vi "Converter.vi"() -> ()   [LabVIEW 2017]
uses:
  CodeElements/SetReturnValue_class/SetReturnValue.lvclass
  E:/Code_Generator/CodeElements/Base/CodeElement.lvclass
  CodeElements/Base/CodeElement.lvclass
panel:
  out "Header":string
  out "Execution":string
  in  "vi path":path
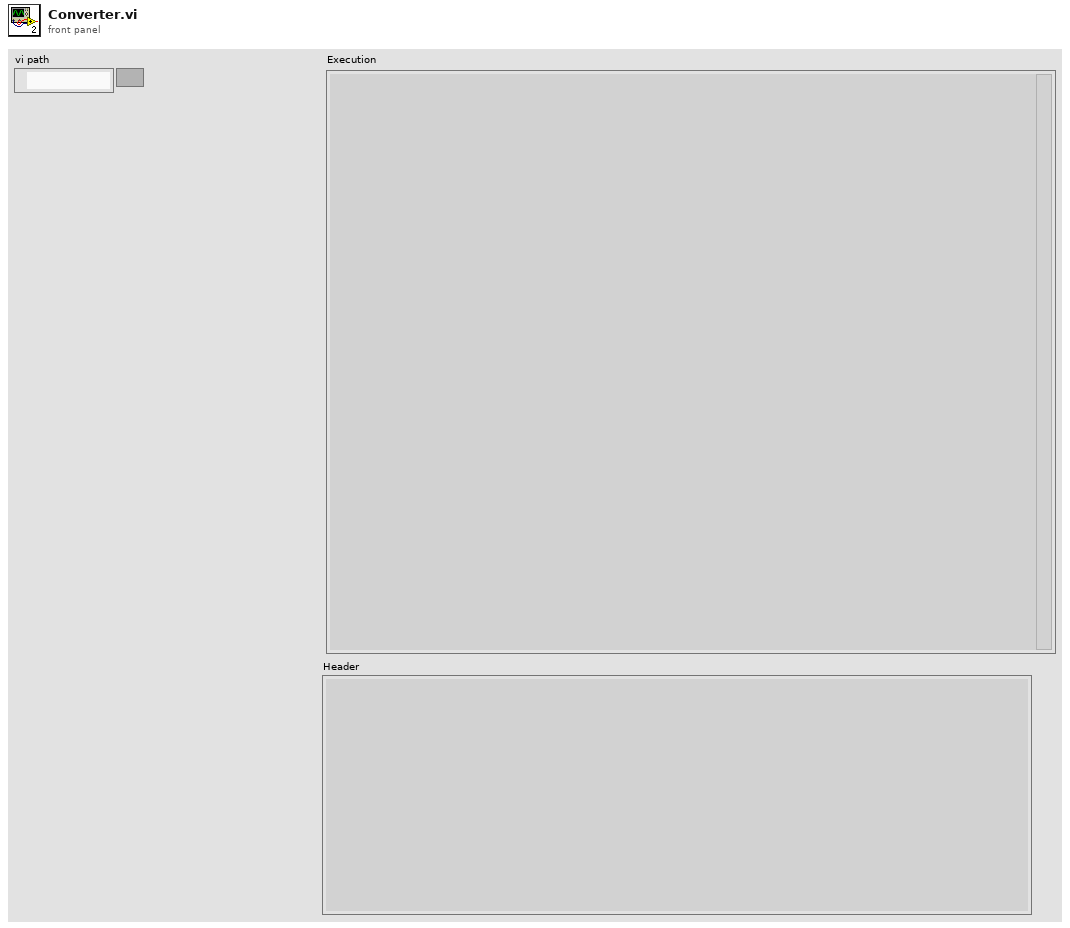
[diagram p1: front panel]
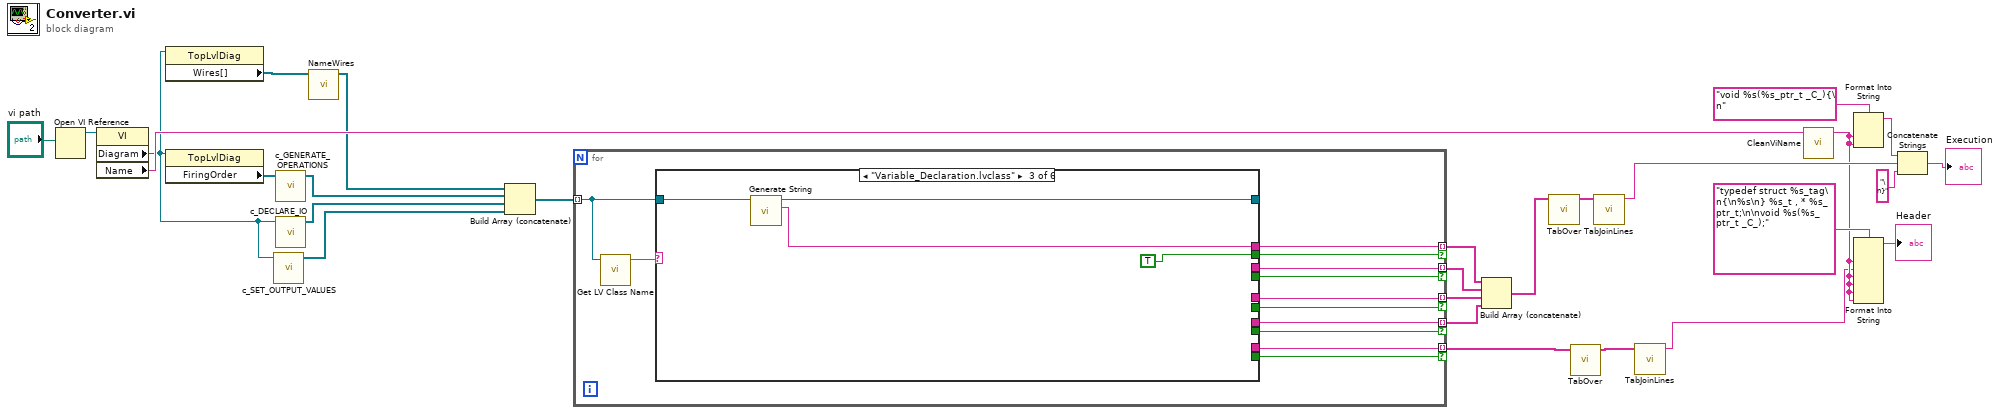
[diagram p0: block diagram]
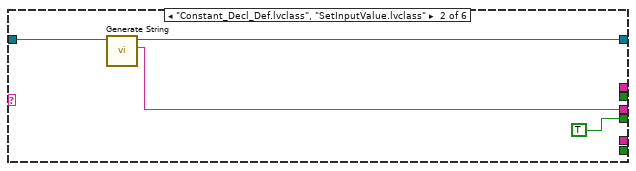
[diagram p3: hidden frame]
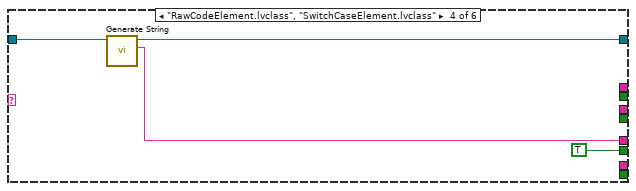
[diagram p4: hidden frame]
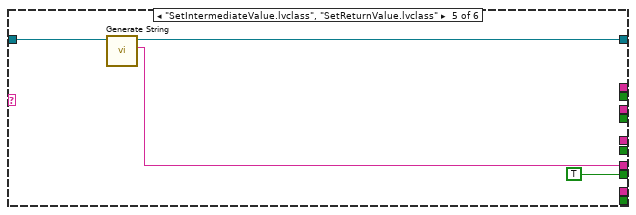
[diagram p5: hidden frame]
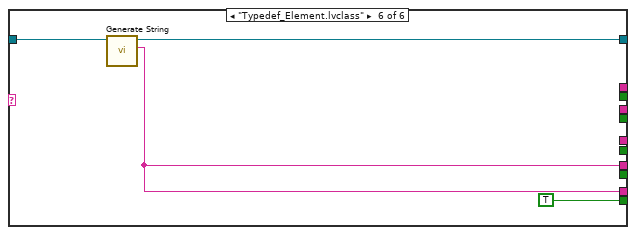
[diagram p6: hidden frame]
diagram:
  n1 = Open VI Reference(vi path="vi path") -> (vi reference=w27:refnum<vi>)  [unwired: 5 in, 1 out]
  n2 = property class="VI"(reference=w27) -> ("Diagram"=w16:refnum<vi>, "Name"=w22:string)  [unwired: 1 in, 2 out]
  n3 = property class="TopLvlDiag"(reference=w16) -> ("Wires[]"=w25:refnum<vi>[])  [unwired: 1 in, 2 out]
  n4 = property class="TopLvlDiag"(reference=w16) -> ("FiringOrder"=w26:refnum<vi>[])  [unwired: 1 in, 2 out]
  n5 = call "c_SET_OUTPUT_VALUES.vi"("TopLevelDiagram in"=w16) -> ("Array"=w12:refnum<class "SetReturnValue.lvclass">[])  [unwired: 10 in]
  n6 = call "c_GENERATE_OPERATIONS.vi"("FiringOrder"=w26) -> ("Array"=w14:refnum<class "CodeElement.lvclass">[])  [unwired: 10 in]
  n7 = call "c_DECLARE_IO.vi"("TopLevelDiagram in"=w16) -> ("CodeElements"=w13:refnum<class "CodeElement.lvclass">[])  [unwired: 10 in]
  n8 = call "NameWires.vi"("Wires[]"=w25) -> ("CodeElements"=w15:refnum<class "CodeElement.lvclass">[])  [unwired: 10 in]
  n9 = Build Array (concatenate)(w15, w14, w13, w12) -> (w11:refnum<class "CodeElement.lvclass">[])
  n10 = for {
    tunnel: w11 -> [w39] mode=indexing
    tunnel: [w38] -> w2 mode=indexing if=w37
    tunnel: [w36] -> w10 mode=indexing if=w35
    tunnel: [w34] -> w9 mode=indexing if=w33
    tunnel: [w32] -> w4 mode=indexing if=w31
    tunnel: [w30] -> w1 mode=indexing if=w29
    n11 = call <vilib>:"Get LV Class Name.vi"("object"=w39) -> ("class name"=w40:string)  [unwired: 9 in, 1 out]
    n12 = case shown="\"Variable_Declaration.lvclass\"" w40 {
      tunnel: [w41 w44 w48 w52 w56 w60] -> _
      tunnel: w39 -> [w41 w45 w49 w53 w57 w61]
      tunnel: [_ w43 _ _ _ _] -> w38
      tunnel: [_ TRUE _ _ _ _] -> w37
      tunnel: [_ _ _ w51 _ _] -> w36
      tunnel: [_ _ _ TRUE _ _] -> w35
      tunnel: [_ _ _ _ TRUE _] -> w33
      tunnel: [_ _ _ _ w54 w59] -> w34
      tunnel: [_ _ _ _ _ w59] -> w32
      tunnel: [_ _ _ _ _ TRUE] -> w31
      tunnel: [_ _ w47 _ _ _] -> w30
      tunnel: [_ _ TRUE _ _ _] -> w29
      frame "False", Default {
      }
      frame "Constant_Decl_Def.lvclass", "SetInputValue.lvclass" {
        n13 = call-dynamic "Generate String.vi"("object in"=w45) -> ("String"=w43:string, "object out"=w44:refnum<class "CodeElement.lvclass">)  [unwired: 8 in, 1 out]
      }
      frame "Variable_Declaration.lvclass" {
        n14 = call-dynamic "Generate String.vi"("object in"=w49) -> ("String"=w47:string, "object out"=w48:refnum<class "CodeElement.lvclass">)  [unwired: 8 in, 1 out]
      }
      frame "RawCodeElement.lvclass", "SwitchCaseElement.lvclass" {
        n15 = call-dynamic "Generate String.vi"("object in"=w53) -> ("String"=w51:string, "object out"=w52:refnum<class "CodeElement.lvclass">)  [unwired: 8 in, 1 out]
      }
      frame "SetIntermediateValue.lvclass", "SetReturnValue.lvclass" {
        n16 = call-dynamic "Generate String.vi"("object in"=w57) -> ("String"=w54:string, "object out"=w56:refnum<class "CodeElement.lvclass">)  [unwired: 8 in, 1 out]
      }
      frame "Typedef_Element.lvclass" {
        n17 = call-dynamic "Generate String.vi"("object in"=w61) -> ("String"=w59:string, "object out"=w60:refnum<class "CodeElement.lvclass">)  [unwired: 8 in, 1 out]
      }
    }
  }
  n18 = Build Array (concatenate)(w1, w2, w10, w9) -> (w6:string[])
  n19 = call "TabOver.vi"("Array in"=w6) -> ("Array out"=w5:string[])  [unwired: 10 in]
  n20 = call "TabOver.vi"("Array in"=w4) -> ("Array out"=w3:string[])  [unwired: 10 in]
  n21 = call "TabJoinLines.vi"("Array"=w5) -> ("String"=w18:string)  [unwired: 10 in]
  n22 = call "TabJoinLines.vi"("Array"=w3) -> ("String"=w8:string)  [unwired: 10 in]
  n23 = call "CleanViName.vi"("Name"=w22) -> ("submatch 1"=w17:string)  [unwired: 10 in]
  n24 = Format Into String(format string="void %s(%s_ptr_t _C_){\n", w17, w17) -> (resulting string=w19:string)  [unwired: 2 in, 1 out]
  n25 = Format Into String(format string="typedef struct %s_tag\n{\n%s\n} %s_t , * %s_ptr_t;\n\nvoid %s(%s_ptr_t _C_);", w17, w8, w17, w17, w17, w17) -> (resulting string=→"Header":string)  [unwired: 2 in, 1 out]
  n26 = Concatenate Strings(w19, w18, "\n}" ("string")) -> (→"Execution":string)
